vi "Test Get Classes Instances.vi"(8 "error in (no error)":errorcluster, 11 "TestCase in":refnum<class "Test Factory Pattern.lvclass">) -> (0 "error out":errorcluster, 3 "TestCase out":refnum<class "Test Factory Pattern.lvclass">)   [LabVIEW 2020, in "Test Factory Pattern.lvclass"]
uses:
  Test Factory Pattern.lvclass
  <vilib>/addons/_JKI Toolkits/VI Tester/TestCase.llb/TestCase.lvclass
  Libraries/Osciloscope Tektronix/Osciloscope Tektronix.lvlib
  C:/Program Files (x86)/National Instruments/LabVIEW 2020/vi.lib/addons/_JKI Toolkits/VI Tester/TestCase.llb/TestCase.lvclass
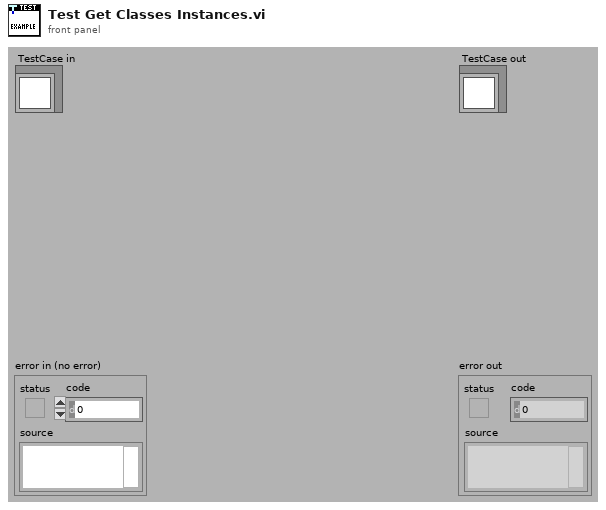
[diagram p1: front panel]
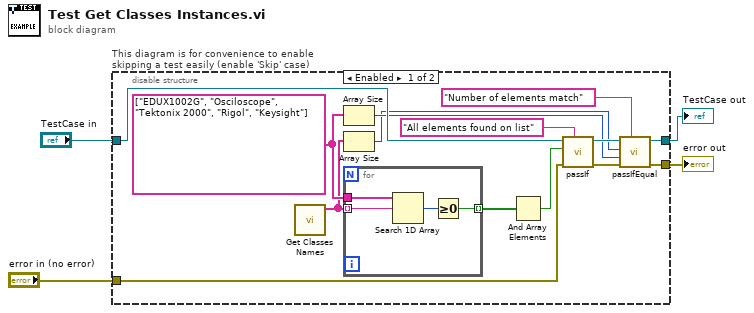
[diagram p0: block diagram]
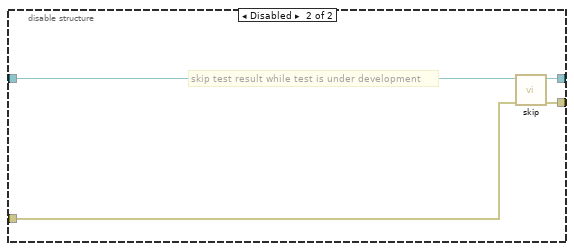
[diagram p2: hidden frame]
diagram:
  n1 = disable-structure "This diagram is for convenience to enable skipping a test easily (enable 'Skip' case)" shown="Enabled" {
    disable-tunnel: "TestCase in" -> [w17 w26]
    disable-tunnel: [w12 w24] -> w1
    disable-tunnel: [w11 w25] -> w3
    disable-tunnel: "error in (no error)" -> [w18 w23]
    frame Enabled {
      w10 = string[] ["EDUX1002G", "Osciloscope", "Tektonix 2000", "Rigol", "Keysight"] ("Classes")
      n2 = call "Get Classes Names.vi"() -> ("Classes"=w8:string[])  [unwired: 11 in]
      n3 = Array Size(array=w10) -> (size(s)=w9:i32)
      n4 = Array Size(array=w8) -> (size(s)=w7:i32)
      n5 = for {
        tunnel: w8 -> [w21] mode=indexing
        tunnel: w10 -> [w22]
        tunnel: [w19] -> w16 mode=indexing
        n6 = Search 1D Array(1D array=w22, element=w21) -> (index of element=w20:i32)  [unwired: 1 in]
        n7 = Greater Or Equal To 0?(x=w20) -> (x >= 0?=w19:bool)
      }
      n8 = And Array Elements(Boolean array=w16) -> (logical AND=w15:bool)
      n9 = call-dynamic "passIf.vi"("custom report message (\"\")"="All elements found on list" ("custom report message (\"\")"), "error in (no error)"=w18, "pass"=w15, "TestCase in"=w17) -> ("error out"=w14:errorcluster, "TestCase out"=w13:refnum<class "Test Factory Pattern.lvclass">)  [unwired: 6 in]
      n10 = call-dynamic "passIfEqual.vi"("custom report message (\"\")"="Number of elements match" ("custom report message (\"\")"), "error in (no error)"=w14, "y"=w9, "x"=w7, "TestCase in"=w13) -> ("error out"=w11:errorcluster, "TestCase out"=w12:refnum<class "Test Factory Pattern.lvclass">)  [unwired: 5 in]
    }
    frame Disabled {
      # "skip test result while test is under development"
      n11 = call <vilib>:"skip.vi"("error in (no error)"=w23, "TestCase in"=w26) -> ("error out"=w25:errorcluster, "TestCase out"=w24:refnum<class "Test Factory Pattern.lvclass">)  [unwired: 8 in]
    }
  }
  "error out" <- w3
  "TestCase out" <- w1
